vi "Collide.vi"(8 "error in (no error)":errorcluster, 9 "angleCorrection in":sgl, 10 "action in":T1, 11 "class data in":refnum<class "Sprite.lvclass">) -> (0 "error out":errorcluster, 3 "class data out":refnum<class "Sprite.lvclass">)   [LabVIEW 2010, in "RenderBase.lvlib" / "Sprite.lvclass"]
doc: "Callback method that is run on collision. This is a basic collision check that implements bouncing."
uses:
  Sprite.lvclass
  SceneObject_class/CollisionAction.ctl
  Sprite.lvclass/Sprite.ctl
  SceneObject_class/SceneObject.lvclass
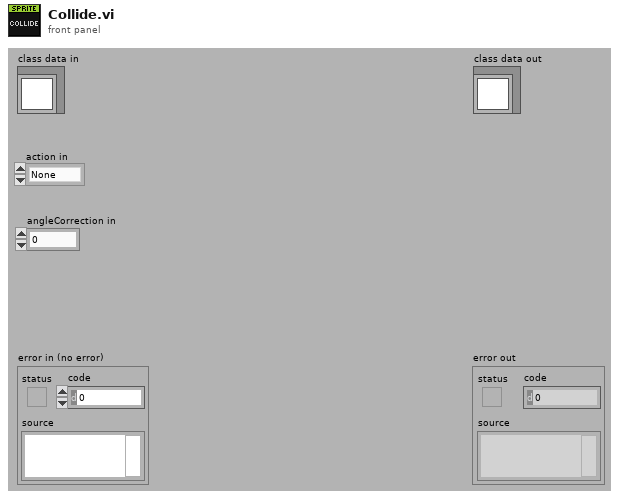
[diagram p1: front panel]
types:
  T1 = typedef "RenderBase.lvlib/SceneObject.lvclass/CollisionAction.ctl" = enum16{"None", "BounceX", "BounceY", "BounceXY"}
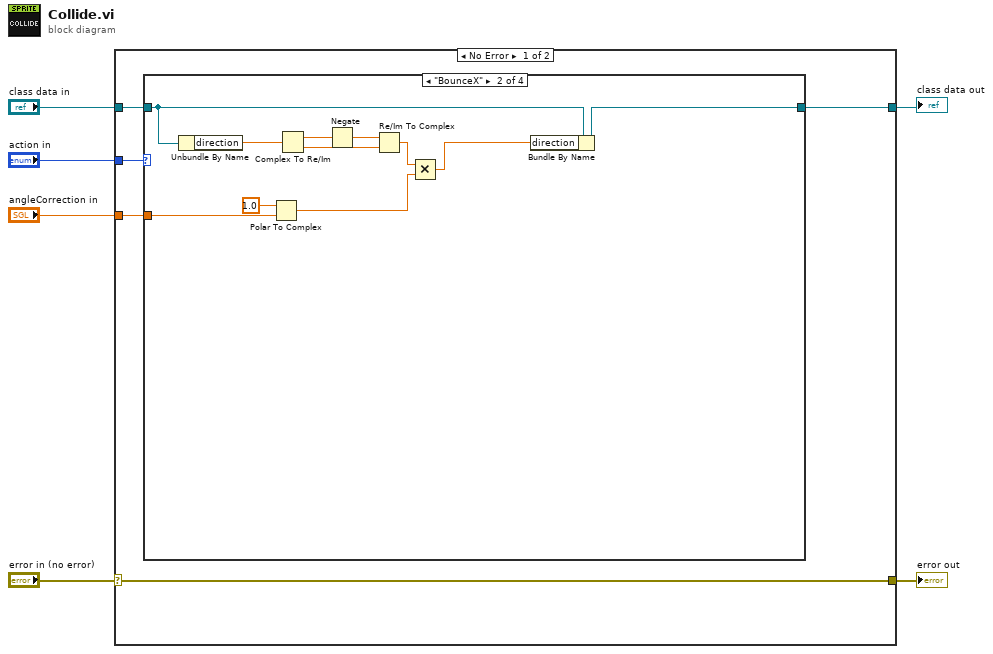
[diagram p0: block diagram]
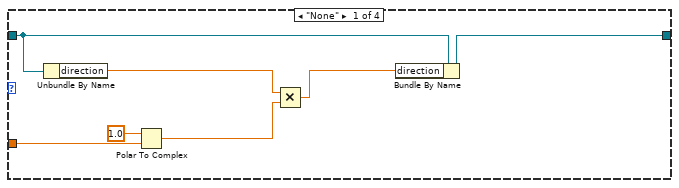
[diagram p2: hidden frame]
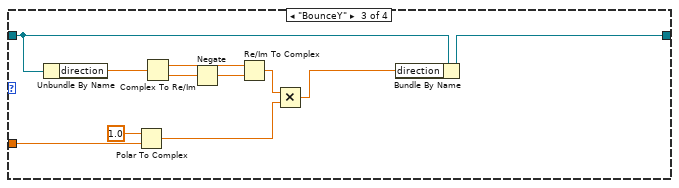
[diagram p3: hidden frame]
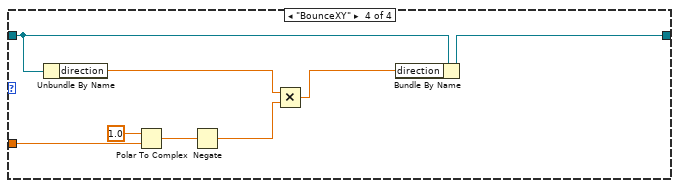
[diagram p4: hidden frame]
diagram:
  n1 = case shown="No Error" "error in (no error)" {
    selector: "error in (no error)" -> [w7 w50]
    tunnel: [w7 w50] -> w5
    tunnel: "class data in" -> [w10 w49]
    tunnel: [w9 w49] -> w3
    tunnel: "action in" -> [w11 _]
    tunnel: "angleCorrection in" -> [w8 _]
    frame No Error {
      n2 = case shown="\"BounceX\"" w11 {
        tunnel: w10 -> [w18 w26 w38 w48]
        tunnel: [w12 w19 w30 w41] -> w9
        tunnel: w8 -> [w17 w24 w37 w47]
        frame "None" {
          n3 = Unbundle By Name(w18) -> ("direction"=w13:csg)
          n4 = Polar To Complex(1:w17, 2:1.0 ("r")) -> (0:w16:cdb)
          n5 = Multiply(x=w13, y=w16) -> (x*y=w14:cdb)
          n6 = Bundle By Name(cluster=w18, "direction"=w14) -> (w12:refnum<class "Sprite.lvclass">)
        }
        frame "BounceX" {
          n7 = Unbundle By Name(w26) -> ("direction"=w21:csg)
          n8 = Polar To Complex(1:w24, 2:sgl 1.0 ("r")) -> (0:w23:csg)
          n9 = Complex To Re/Im(x + iy=w21) -> (x=w29:sgl, y=w28:sgl)
          n10 = Negate(x=w29) -> (-x=w25:sgl)
          n11 = Re/Im To Complex(1:w28, 2:w25) -> (0:w27:csg)
          n12 = Multiply(x=w27, y=w23) -> (x*y=w20:csg)
          n13 = Bundle By Name(cluster=w26, "direction"=w20) -> (w19:refnum<class "Sprite.lvclass">)
        }
        frame "BounceY" {
          n14 = Unbundle By Name(w38) -> ("direction"=w31:csg)
          n15 = Polar To Complex(1:w37, 2:1.0 ("r")) -> (0:w36:cdb)
          n16 = Complex To Re/Im(x + iy=w31) -> (x=w33:sgl, y=w40:sgl)
          n17 = Negate(x=w40) -> (-x=w34:sgl)
          n18 = Re/Im To Complex(1:w34, 2:w33) -> (0:w39:csg)
          n19 = Multiply(x=w39, y=w36) -> (x*y=w32:cdb)
          n20 = Bundle By Name(cluster=w38, "direction"=w32) -> (w30:refnum<class "Sprite.lvclass">)
        }
        frame "BounceXY" {
          n21 = Unbundle By Name(w48) -> ("direction"=w43:csg)
          n22 = Polar To Complex(1:w47, 2:1.0 ("r")) -> (0:w46:cdb)
          n23 = Negate(x=w46) -> (-x=w44:cdb)
          n24 = Multiply(x=w43, y=w44) -> (x*y=w42:cdb)
          n25 = Bundle By Name(cluster=w48, "direction"=w42) -> (w41:refnum<class "Sprite.lvclass">)
        }
      }
    }
    frame Error {
    }
  }
  "error out" <- w5
  "class data out" <- w3
